vi "Compute Destination Endpoints.vi"(8 "error in":errorcluster, 9 "endpoints":string[](array[string]), 10 "source endpoint":string, 11 "instrument handle in":refnum<k15>) -> (0 "error out":errorcluster, 2 "possible destinations":string[](array[string]), 3 "instrument handle out":refnum<k15>)   [LabVIEW 2017, in "NI-SWITCH Scripting.lvlib"]
uses:
  NI-SWITCH Scripting.lvlib
  <instrlib>/niSwitch/niSwitch.llb/niSwitch Path Capability.ctl
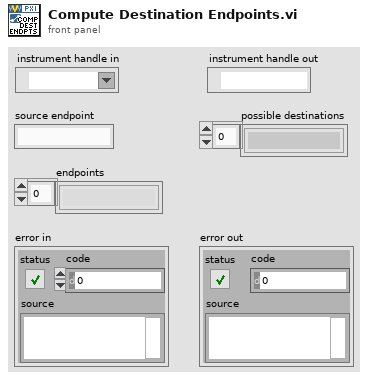
[diagram p1: front panel]
types:
  T1 = typedef "niSwitch Path Capability.ctl" = i32
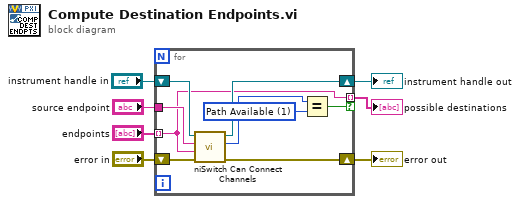
[diagram p0: block diagram]
diagram:
  n1 = for {
    tunnel: "endpoints" -> [w10] mode=indexing
    shift-right: [w15] -> w5
    shift-left: "error in" -> [w16]
    shift-right: [w13] -> w1
    shift-left: "instrument handle in" -> [w14]
    tunnel: "source endpoint" -> [w12]
    tunnel: [w10] -> w7 mode=indexing if=w9
    w8 = T1 1 items=["Path Available"=1, "Path Exists"=2, "Path Unsupported"=3, "Resource in Use"=4, "Source Conflict"=5, "Channel Not Available"=6] ("path capability")
    n2 = call <instrlib>:"niSwitch Can Connect Channels.vi"("error in (no error)"=w16, "channel 2"=w10, "channel 1"=w12, "instrument handle"=w14) -> ("error out"=w15:errorcluster, "path capability"=w11:T1, "instrument handle out"=w13:refnum<k15>)  [unwired: 5 in]
    n3 = Equal?(x=w11, y=w8) -> (x = y?=w9:bool)
  }
  "possible destinations" <- w7
  "error out" <- w5
  "instrument handle out" <- w1
